vi "UI_page13.vi"(10 "传递队列输入":refnum<queue>, 11 "notifier":refnum<notifier>) -> ()   [LabVIEW 2012]
uses:
  <vilib>/Utility/miscctls.llb/LVDateTimeRec.ctl
  <vilib>/GPower/VIRegister/Library/Convert/ToBool.vi
  <vilib>/GPower/VIRegister/Library/Convert/ToU32.vi
  <vilib>/GPower/VIRegister/Library/Convert/ToU8.vi
  <vilib>/GPower/VIRegister/Library/SubVIs/FindRegisterData.vi
  <vilib>/GPower/VIRegister/Library/SubVIs/ReadSub.vi
  <vilib>/GPower/VIRegister/Library/SubVIs/WriteSub.vi
  <vilib>/GPower/Error/Library/FilterCodes.vi
  <vilib>/GPower/Error/Library/Filter/FilterMulti.vi
  <vilib>/GPower/VIRegister/Library/QManager/GetRegisterData.vi
  <vilib>/GPower/Error/Library/SetError.vi
  <vilib>/GPower/Error/Library/SplitAppended.vi
  <vilib>/GPower/VIRegister/Library/QManager/QManagerAction.vi
  <vilib>/GPower/Error/Library/ErrorType.vi
  <vilib>/GPower/Error/Library/SubVIs/ExplanationToError.vi
  <vilib>/GPower/VIRegister/Library/QManager/GetQName.vi
  <vilib>/GPower/VIRegister/Library/QManager/StartQManager.vi
  <vilib>/Utility/error.llb/Trim Whitespace.vi
  <vilib>/dlg_ctls.llb/Space Constant.vi
  <vilib>/Utility/error.llb/Error Code Database.vi
  <vilib>/GPower/Error/Library/SubVIs/SetStatus.vi
  <vilib>/GPower/Error/Library/AppendErrors.vi
  <vilib>/GPower/Error/Library/Append/AppendSingle.vi
  <vilib>/GPower/VIRegister/VIRegister.lvlib
  <vilib>/measure/NI_MABase.lvlib
panel:
  out "试验已用时":timestamp=timestamp(-28800 s since 1904-01-01) format="%<%H:%M:%S>T"
  in  "测试时间设定":timestamp=timestamp(-28800 s since 1904-01-01) format="%<%H:%M:%S>T"
  in  "停止测量":bool
  in  "开始测量":bool
  out "温度":string
  out "脉冲计数":string
  out "主份G3陀螺脉冲计数":dbl(graph)
  out "主份A3加速度计脉冲计数":dbl(graph)
  out "主份G2陀螺脉冲数":dbl(graph)
  out "主份A2加速度计脉冲计数":dbl(graph)
  out "主份G1陀螺脉冲数":dbl(graph)
  out "主份A1加速度计脉冲计数":dbl(graph)
  out "正确帧计数":u16
  out "错误帧计数":u32
  in  "加计大小量程":enum32{"小量程", "大量程"}(radio)=enum."大量程"
  in  "穿插错误":bool
  in  "少数据字":bool
  in  "少验和":bool
  in  "少帧头":bool
  in  "验和错":bool
  in  "帧头错":bool
  in  "无数据":bool
  in  "地检按钮":bool
  in  "加表频率":dbl=1.0 min=0.1 max=10.0 step=0.1
  in  "加表幅值":dbl=1.0
  in  "陀螺频率":dbl=1.0 min=0.1 max=10.0 step=0.1
  in  "陀螺幅值":dbl=1.0
  # "备  份"
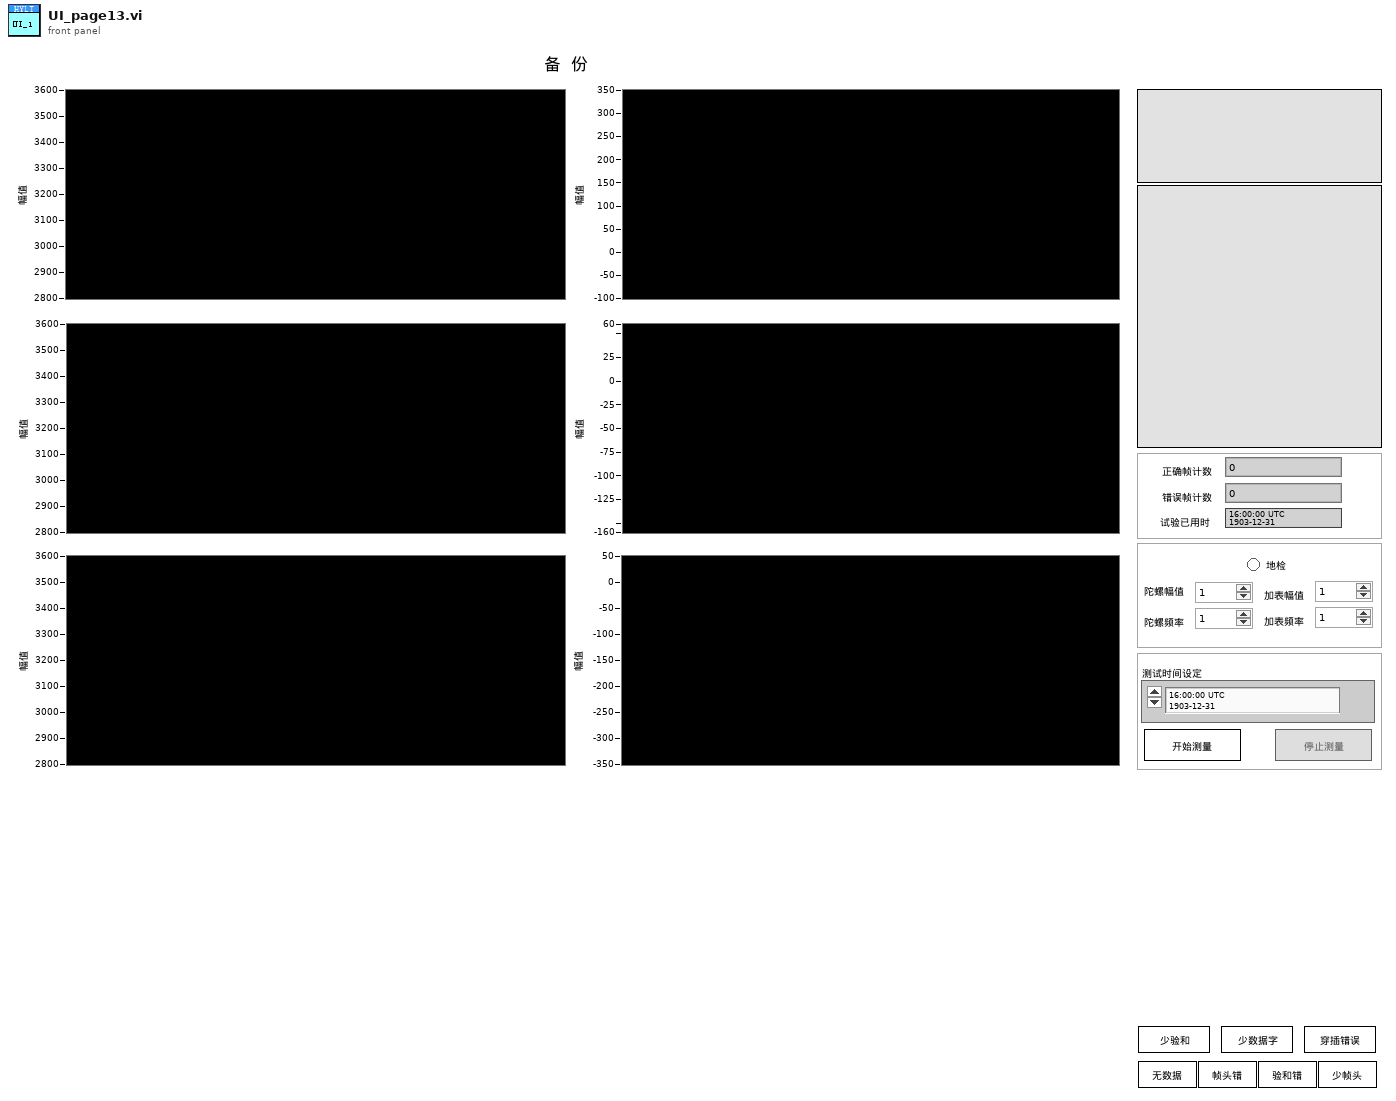
[diagram p1: front panel]
types:
  T1 = typedef "LVDateTimeRec.ctl" = cluster{"fractional second":dbl, "second":i32, "minute":i32, "hour":i32, "day of month":i32, "month":i32, "year":i32, "day of week":i32, "day of year":i32, "DST":i32}
  T2 = enum8{"Enabled", "Disabled", "Disabled and Grayed Out"}
  T3 = enum32{"invalid app kind", "Development System", "Run Time System", "Student Edition", "Embedded LabVIEW", "Evaluation", "Custom"}
  T4 = enum32{"Invalid", "Standard", "Closed", "Hidden", "Minimized", "Maximized"}
  T5 = cluster{"Core":cluster{"Current VI Reference":refnum<vi>, "Close Panel on Exit?":bool}, "传递队列输入":refnum<queue>, "信息帧":cluster{" 数据帧名称":string, " 数据":string, "备用操作符":bool, "起始地址":i32, "读写标志":i32, "长度":i32}, "主份控制指令":u16, "备份控制指令":u16, "notifier ":refnum<notifier>, "秒计数":i64, "起始时间":i64, "定时控制":bool}
  T6 = cluster{" 数据帧名称":string, " 数据":string, "备用操作符":bool, "起始地址":i32, "读写标志":i32, "长度":i32}
  T7 = cluster{"Current VI Reference":refnum<vi>, "Close Panel on Exit?":bool}
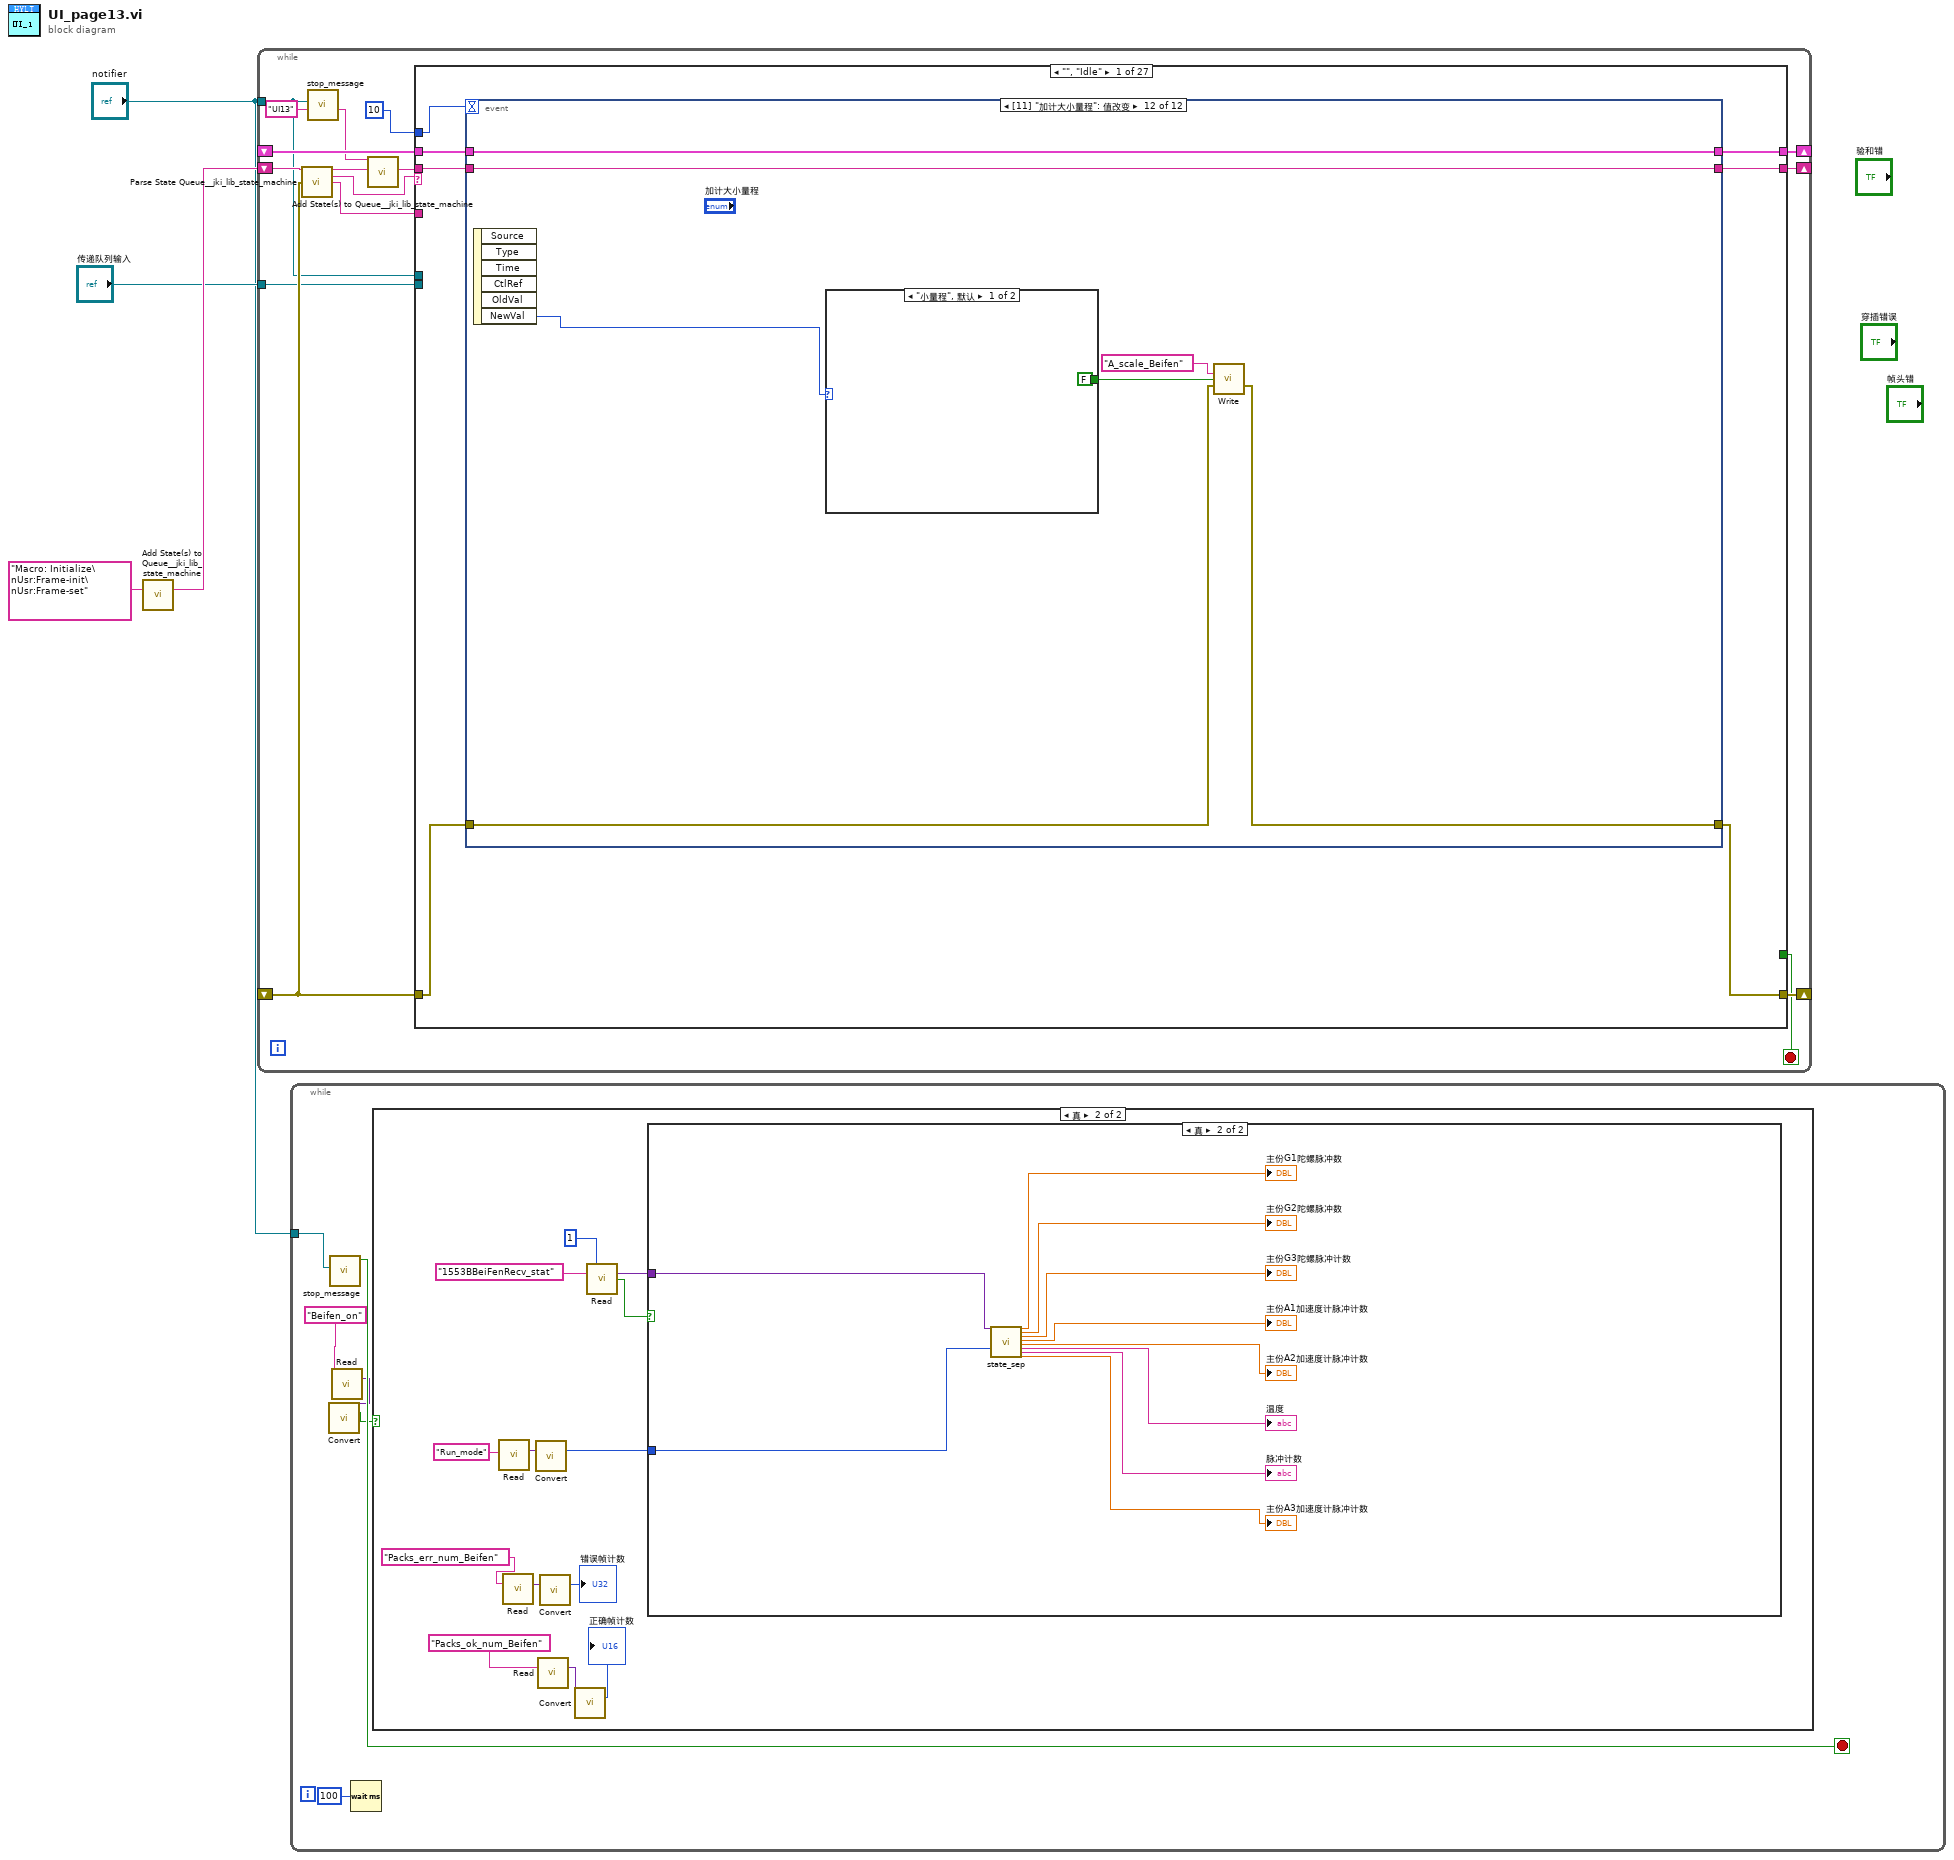
[diagram p0: block diagram]
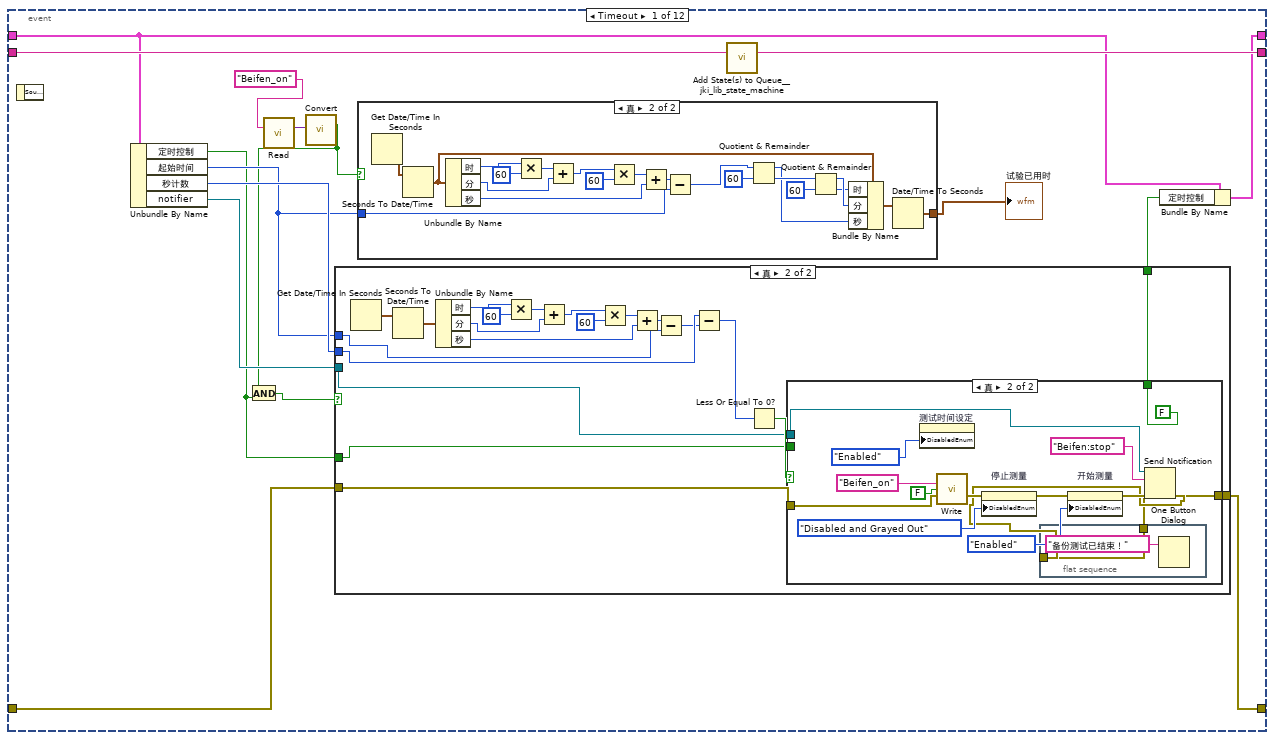
[diagram p4: hidden frame]
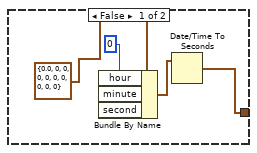
[diagram p5: hidden frame]
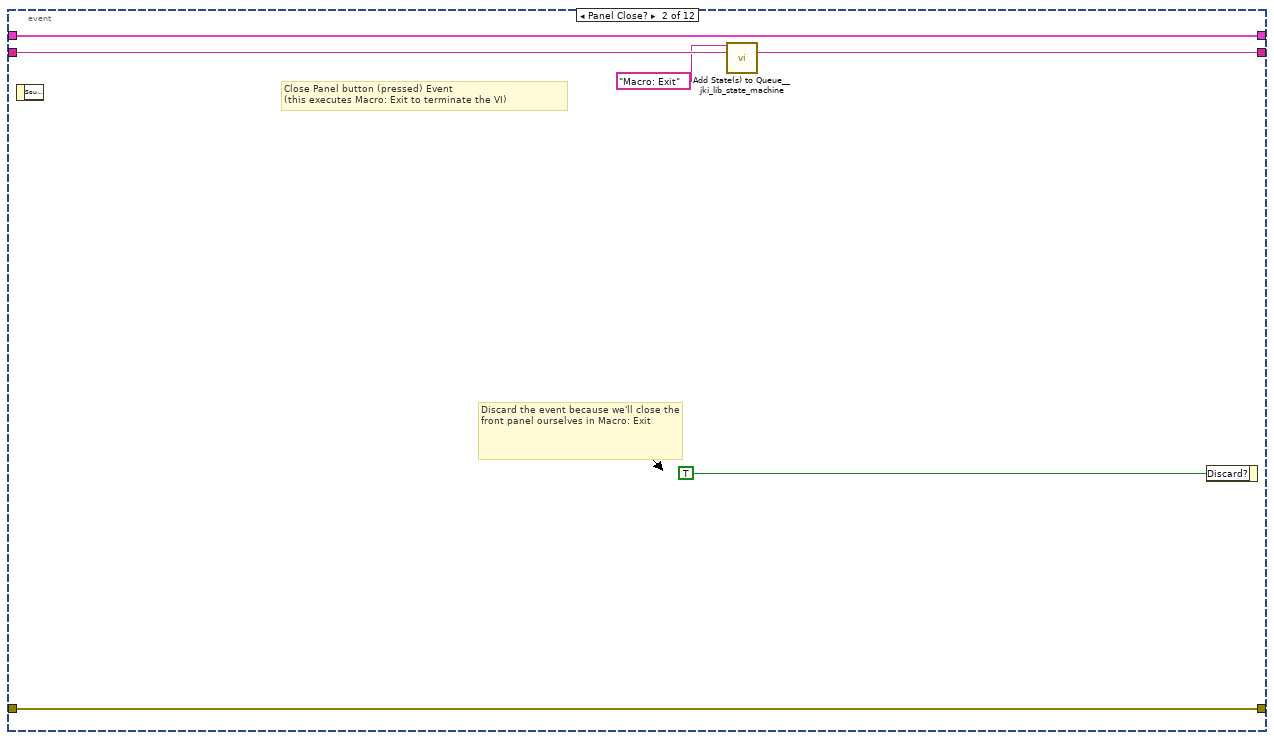
[diagram p8: hidden frame]
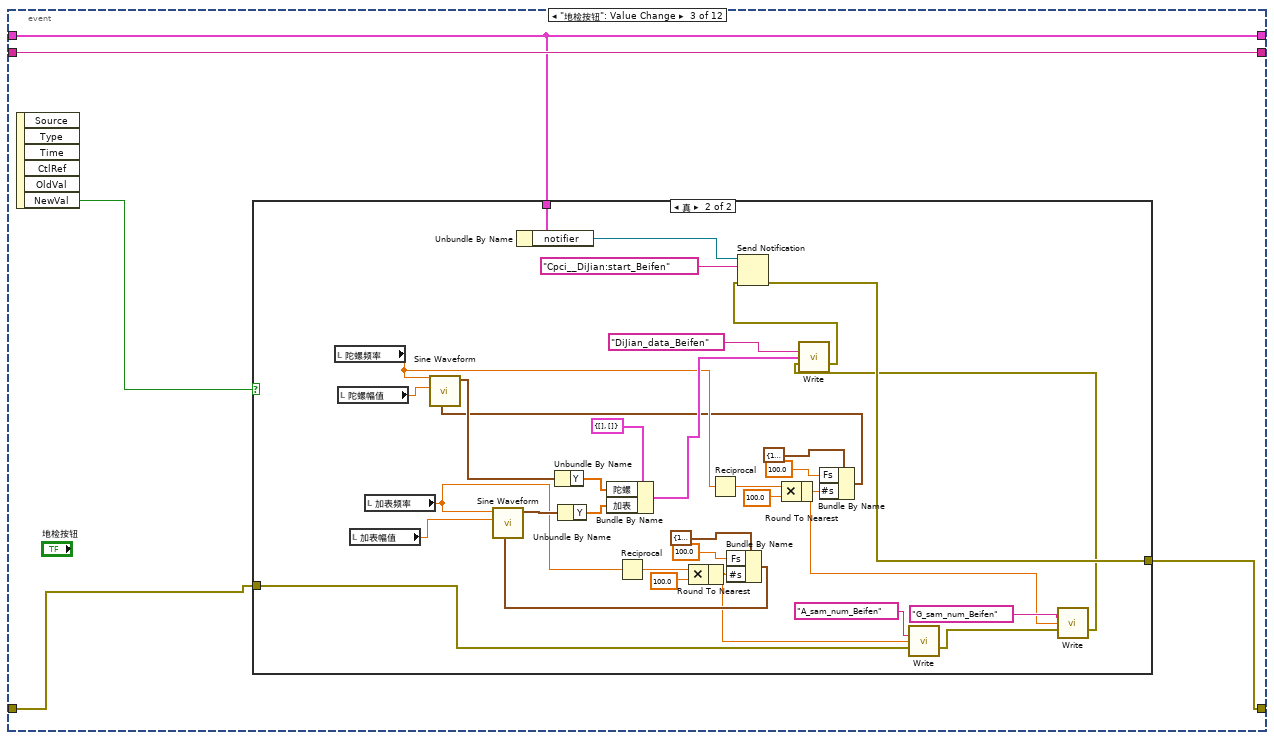
[diagram p9: hidden frame]
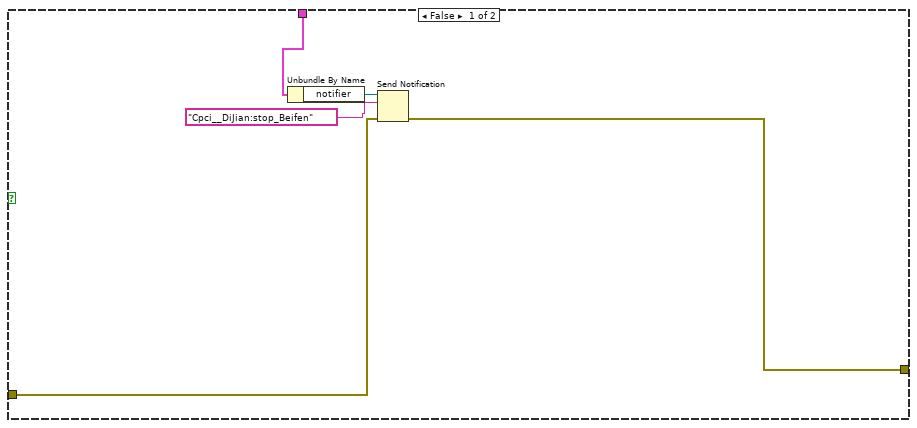
[diagram p10: hidden frame]
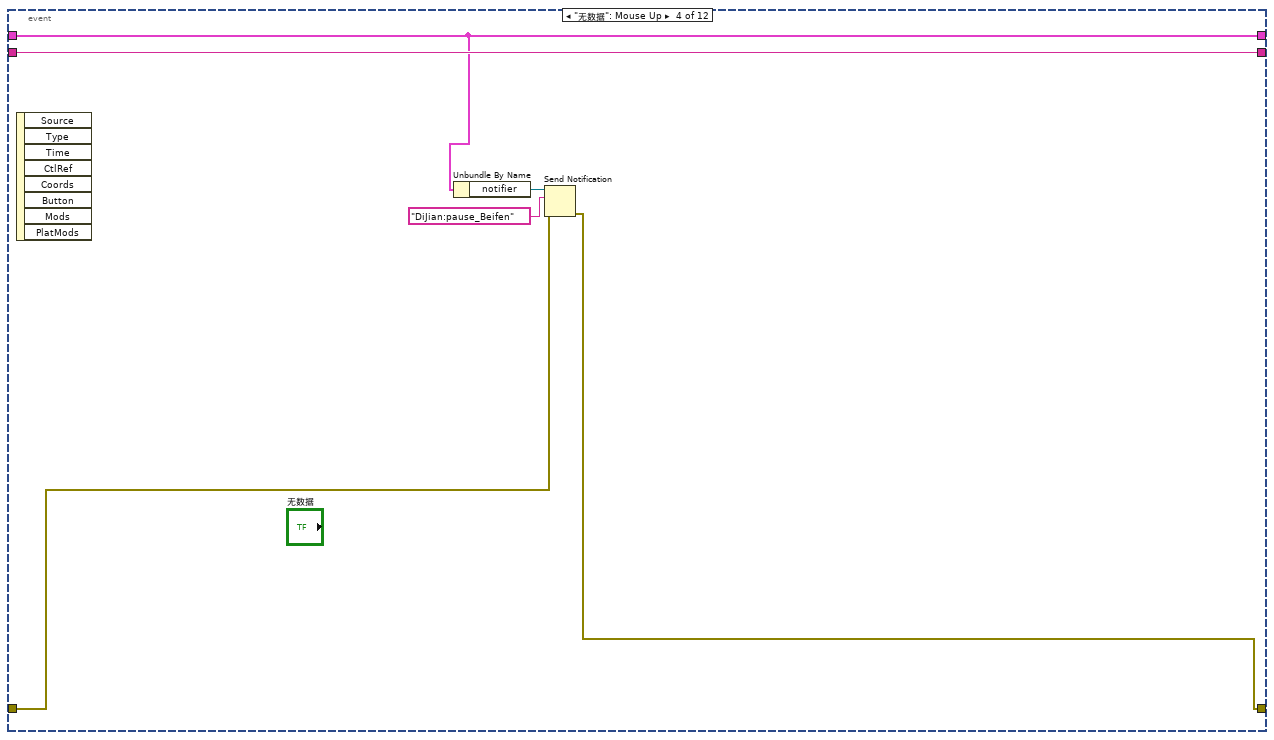
[diagram p11: hidden frame]
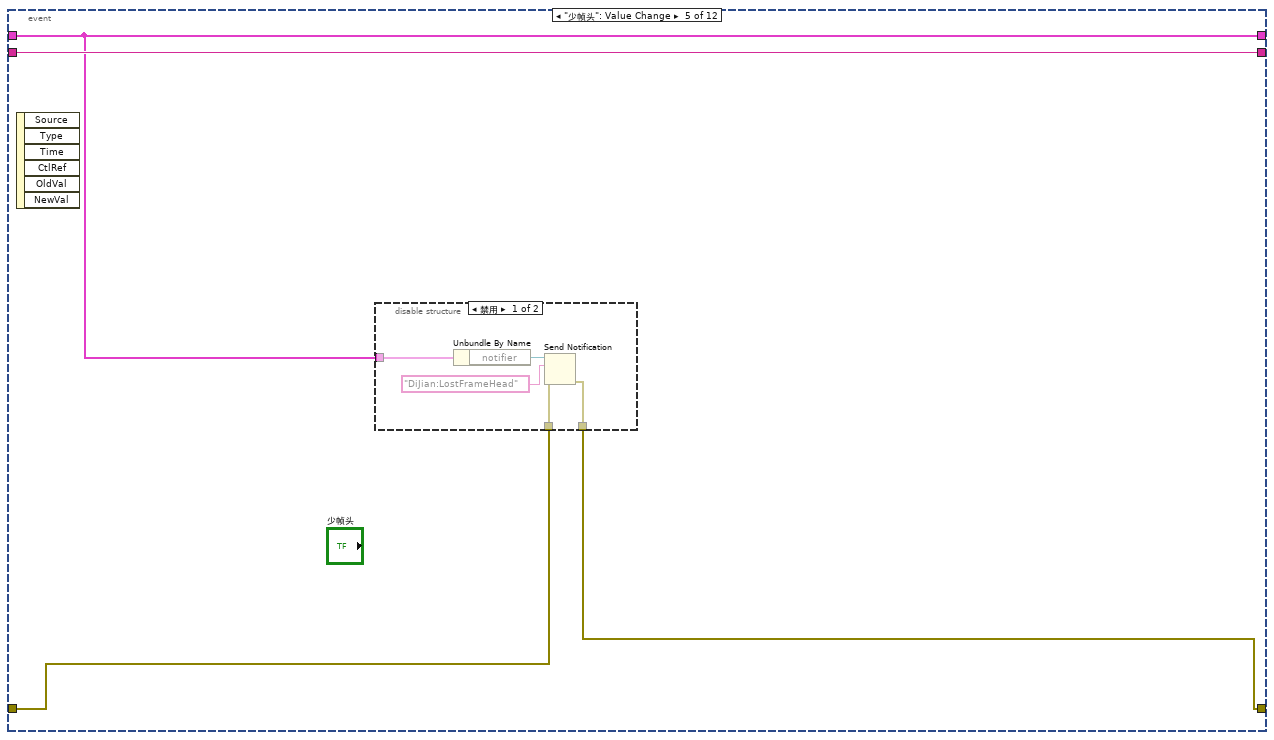
[diagram p12: hidden frame]
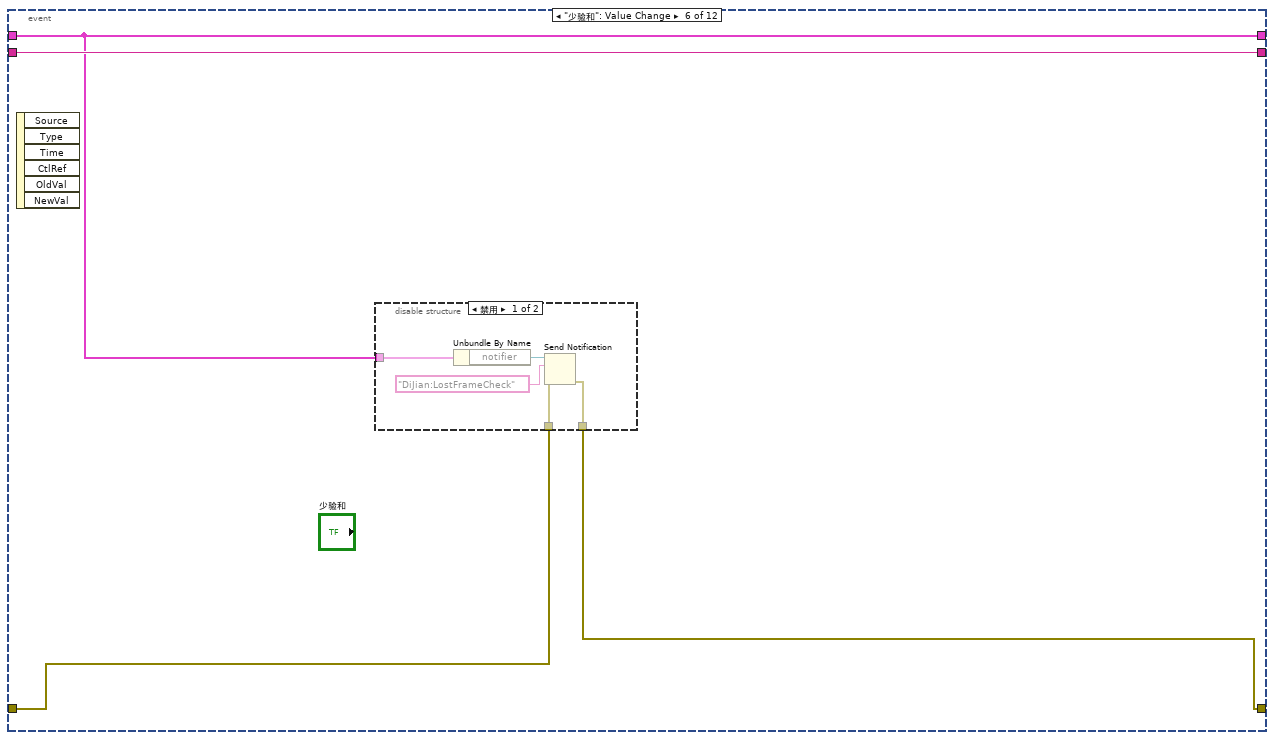
[diagram p14: hidden frame]
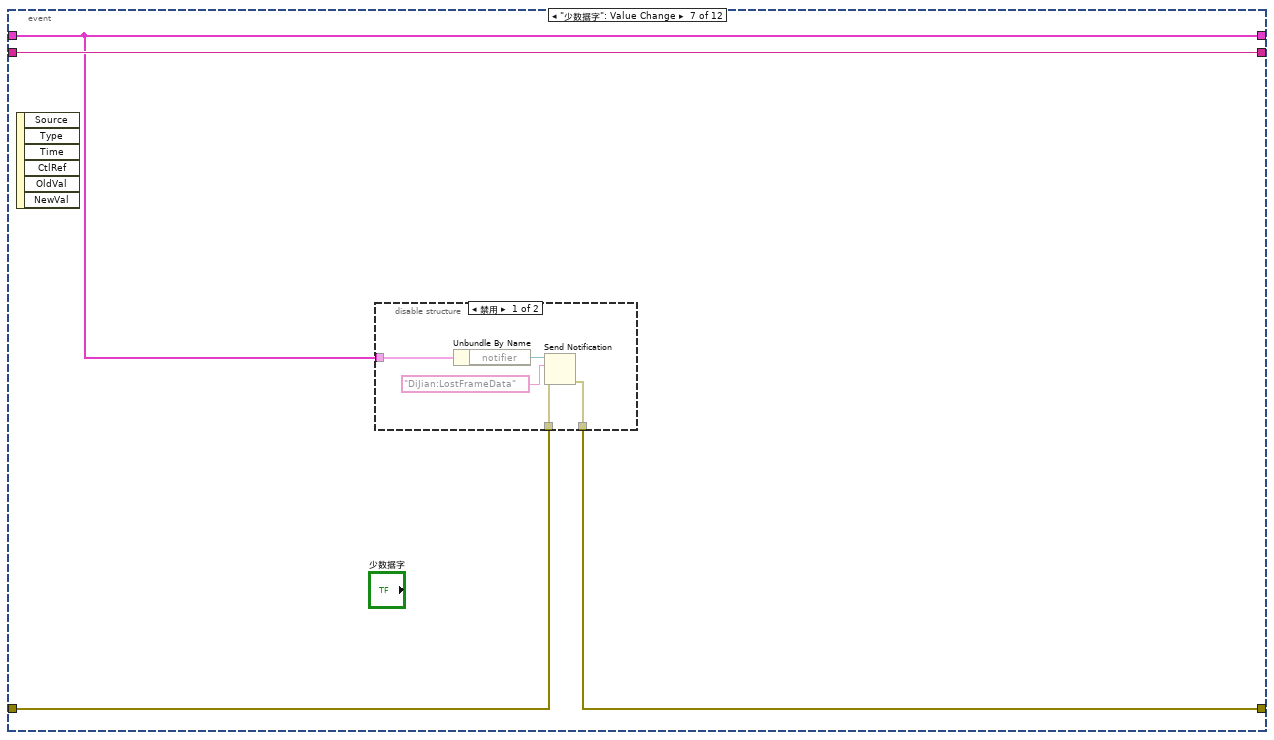
[diagram p16: hidden frame]
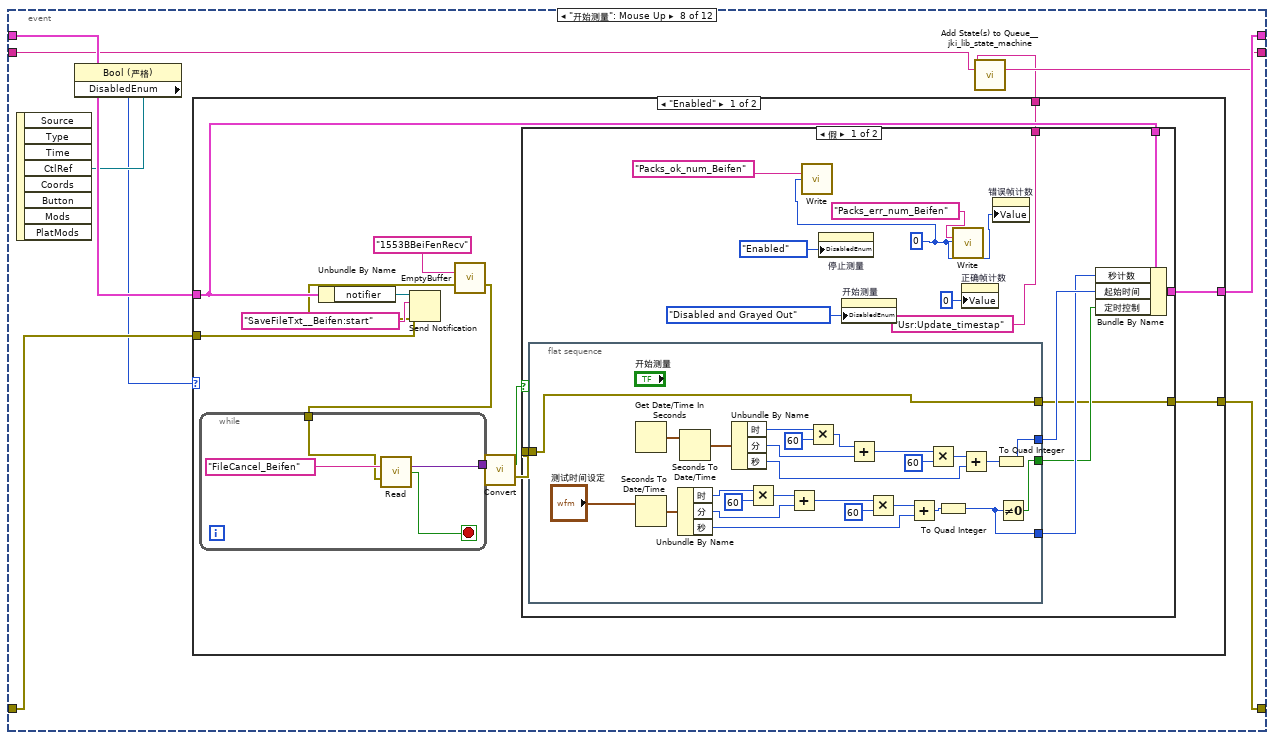
[diagram p18: hidden frame]
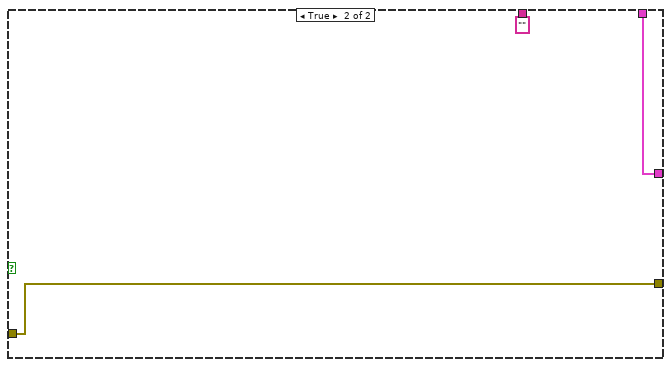
[diagram p19: hidden frame]
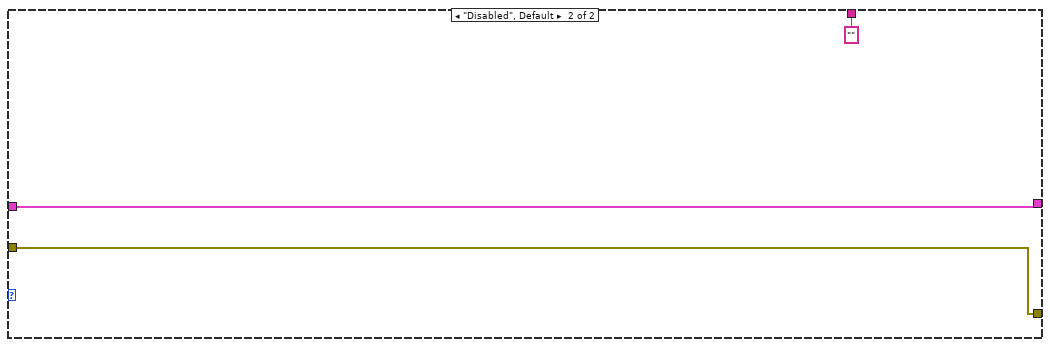
[diagram p20: hidden frame]
diagram:
  n1 = call <vilib>:"Add State(s) to Queue__jki_lib_state_machine.vi"("State(s) in (\"\")"="Macro: Initialize\nUsr:Frame-init\nUsr:Frame-set") -> ("States Out"=w4:string)  [unwired: 14 in]
  n2 = while "JKI - String-Based Queued State Machine (Basic) v1.0" {
    shift-right: [w14] -> _
    shift-left: _ -> [w13]
    shift-right: [w17] -> _
    shift-left: _ -> [w11]
    shift-right: [w16] -> _
    shift-left: w4 -> [w18]
    tunnel: "notifier" -> [w6]
    tunnel: "传递队列输入" -> [w7]
    stop <- w15 stop-if-true
    n3 = call <vilib>:"Parse State Queue__jki_lib_state_machine.vi"("State Queue"=w18, "Error In (no error)"=w11) -> ("Remaining States"=w10:string, "Current State"=w20:string, "Arguments"=w19:string)  [unwired: 11 in]
    n4 = call "stop_message.vi"("识别符"="UI13", "notifier"=w6) -> ("通知"=w9:string)  [unwired: 8 in, 1 out]
    n5 = call <vilib>:"Add State(s) to Queue__jki_lib_state_machine.vi"("State(s) in Front (\"\")"=w9, "State(s) in (\"\")"=w10) -> ("States Out"=w8:string)  [unwired: 13 in]
    n6 = case shown="\"\", \"Idle\"" w20 {
      selector: w20 -> [_ _ w353 _ _ _ _ _ _ _ _ _ _ _ _ _ _ _ _ _ _ _ _ _ _ _ _]
      tunnel: w8 -> [w21 w352 w357 w375 w381 w386 w390 w406 w412 w416 w425 w431 w441 w473 w478 w488 w492 w499 w519 w539 w558 w584 w600 w605 w610 w622 w640]
      tunnel: w19 -> [_ _ _ _ _ _ _ _ _ _ _ w426 w436 _ _ _ _ w493 w513 w533 _ _ _ _ _ _ _]
      tunnel: w13 -> [w26 w349 w355 w366 w378 w384 w387 _ w407 w413 w423 w429 w437 w470 w475 w485 w489 w497 w517 w537 w556 w582 w597 w602 w607 w618 w627]
      tunnel: [w25 w350 w359 w372 errorcluster {"status"=FALSE, "code"=0, "source"=""} ("error out") w383 w388 w403 w408 w414 w422 w427 w438 w471 w476 w486 w490 w495 w515 w535 w554 w580 w598 w603 w608 w620 w625] -> w17
      tunnel: w11 -> [w24 w350 w358 w372 w377 w383 w388 w403 w409 w414 w422 w428 w439 w471 w476 w486 w490 w496 w516 w536 w555 w581 w598 w603 w608 w620 w625]
      tunnel: [w27 w351 w356 w374 w380 w385 w389 w405 w411 w415 w424 w430 w440 w472 w477 w487 w491 w498 w518 w538 w557 w583 w599 w604 w609 w621 w639] -> w16
      tunnel: [_ _ _ _ _ TRUE _ _ _ _ _ _ _ _ _ _ _ _ _ _ _ _ _ _ _ _ _] -> w15
      tunnel: [w23 w349 w355 w373 w378 w384 w387 w404 w407 w413 w423 w429 w437 w470 w475 w485 w489 w494 w514 w534 w553 w579 w597 w602 w606 w618 w626] -> w14
      tunnel: 10 ("Timeout") -> [w22 _ _ _ _ _ _ _ _ _ _ _ _ _ _ _ _ _ _ _ _ _ _ _ _ _ _]
      tunnel: w7 -> [_ _ _ _ _ _ _ w400 _ _ _ _ _ _ _ _ _ _ _ _ _ _ _ _ _ _ _]
      tunnel: w6 -> [_ _ _ _ _ _ _ w396 _ _ _ _ _ _ _ _ _ _ _ _ _ _ _ _ _ _ _]
      frame "", "Idle" {
        n7 = event shown="[11] \"加计大小量程\": 值改变" {
          selector: _ -> [_ _ _ _ _ _ _ _ _ _ _ _]
          dyn-events: _ -> [_ _ _ _ _ _ _ _ _ _ _ _]
          timeout: w22 -> [_ _ _ _ _ _ _ _ _ _ _ _]
          tunnel: w21 -> [w43 w115 w120 w166 w170 w179 w188 w196 w272 w307 w338 w340]
          tunnel: [w42 w114 w120 w166 w170 w179 w188 w195 w272 w307 w338 w340] -> w27
          tunnel: w26 -> [w37 w112 w119 w165 w169 w178 w187 w201 w269 w294 w339 w341]
          tunnel: [w38 w113 w117 w163 w167 w176 w185 w199 w270 w306 w335 w342] -> w25
          tunnel: w24 -> [w39 w113 w118 w164 w168 w177 w186 w202 w271 w306 w334 w343]
          tunnel: [w36 w112 w119 w165 w169 w178 w187 w200 w268 w293 w339 w341] -> w23
          event Timeout {
            n8 = event-data() -> ()  [unwired: 1 in, 1 out]
            n9 = Unbundle By Name(w37) -> ("定时控制"=w28:bool, "起始时间"=w34:i64, "秒计数"=w41:i64, "notifier"=w40:refnum<notifier>)
            n10 = call <vilib>:"Read.vi"("Register name"="Beifen_on") -> ("Register value"=w31:variant)  [unwired: 11 in, 3 out]
            n11 = call-poly <vilib>:"Convert.vi"("Register value in"=w31) -> ("Register value out"=w30:bool)  [unwired: 13 in, 1 out]
            n12 = And(x=w30, y=w28) -> (x .and. y?=w29:bool)
            n13 = case shown="真" w29 {
              tunnel: w34 -> [_ w82]
              tunnel: w41 -> [_ w81]
              tunnel: w40 -> [_ w75]
              tunnel: w39 -> [w70 w74]
              tunnel: [w70 w73] -> w38
              tunnel: [w69 w72] -> w35
              tunnel: w28 -> [w69 w71]
              frame False {
              }
              frame True {
                n14 = Get Date/Time In Seconds() -> (seconds since 1Jan1904=w78:timestamp)
                n15 = Seconds To Date/Time(time stamp (now)=w78) -> (date time rec=w79:T1)  [unwired: 1 in]
                n16 = Unbundle By Name(w79) -> ("时"=w84:i32, "分"=w87:i32, "秒"=w91:i32)
                n17 = Multiply(x=w84, y=60) -> (x*y=w86:i32)
                n18 = Add(x=w86, y=w87) -> (x+y=w88:i32)
                n19 = Multiply(x=w88, y=60) -> (x*y=w90:i32)
                n20 = Add(x=w90, y=w91) -> (x+y=w83:i32)
                n21 = Subtract(x=w83, y=w82) -> (x-y=w80:i64)
                n22 = Subtract(x=w81, y=w80) -> (x-y=w77:i64)
                n23 = Less Or Equal To 0?(x=w77) -> (x <= 0?=w76:bool)
                n24 = case shown="真" w76 {
                  tunnel: w75 -> [_ w99]
                  tunnel: w74 -> [w93 w98]
                  tunnel: [w93 w94] -> w73
                  tunnel: [w92 FALSE] -> w72
                  tunnel: w71 -> [w92 _]
                  frame False {
                  }
                  frame True {
                    n25 = property on="测试时间设定" class="AbsTime (严格)"("DisabledEnum"=T2."Enabled" ("禁用")) -> ()  [unwired: 2 in, 2 out]
                    n26 = call <vilib>:"Write.vi"("Register name"="Beifen_on", "Register value"=FALSE ("停止测量"), "Error in"=w98) -> ("Error out"=w101:errorcluster)  [unwired: 10 in, 2 out]
                    n27 = property on="停止测量" class="Bool (严格)"(error in=w101, "DisabledEnum"=T2."Disabled and Grayed Out" ("禁用")) -> (error out=w102:errorcluster)  [unwired: 1 in, 1 out]
                    n28 = flat-sequence {
                      tunnel: w95 -> [w108]
                      tunnel: [w108] -> w94
                      frame #0 {
                        n29 = One Button Dialog(message="备份测试已结束！" ("消息")) -> ()  [unwired: 1 in, 1 out]
                      }
                    }
                    n30 = property on="开始测量" class="Bool (严格)"(error in=w102, "DisabledEnum"=T2."Enabled" ("禁用")) -> (error out=w100:errorcluster)  [unwired: 1 in, 1 out]
                    n31 = Send Notification(notification="Beifen:stop" ("通知"), notifier=w99, error in (no error)=w100) -> (error out=w95:errorcluster)  [unwired: 1 out]
                  }
                }
              }
            }
            n32 = case shown="真" w30 {
              tunnel: w34 -> [_ w58]
              tunnel: [w44 w50] -> w33
              frame False {
                w46 = 0 ("时")
                n33 = Bundle By Name(cluster=T1 {"fractional second"=0.0, "second"=0, "minute"=0, "hour"=0, "day of month"=0, "month"=0, "year"=0, "day of week"=0, "day of year"=0, "DST"=0} ("日期时间记录 2"), "hour"=w46, "minute"=w46, "second"=w46) -> (w47:T1)
                n34 = Date/Time To Seconds(2:w47) -> (0:w44:timestamp)  [unwired: 1 in]
              }
              frame True {
                n35 = Get Date/Time In Seconds() -> (seconds since 1Jan1904=w68:timestamp)
                n36 = Seconds To Date/Time(time stamp (now)=w68) -> (date time rec=w51:T1)  [unwired: 1 in]
                n37 = Unbundle By Name(w51) -> ("时"=w66:i32, "分"=w63:i32, "秒"=w59:i32)
                n38 = Multiply(x=w66, y=60) -> (x*y=w64:i32)
                n39 = Add(x=w64, y=w63) -> (x+y=w62:i32)
                n40 = Multiply(x=w62, y=60) -> (x*y=w60:i32)
                n41 = Add(x=w60, y=w59) -> (x+y=w67:i32)
                n42 = Subtract(x=w67, y=w58) -> (x-y=w48:i64)
                n43 = Quotient & Remainder(x=w48, y=60) -> (x-y*floor(x/y)=w49:i64, floor(x/y)=w53:i64)
                n44 = Quotient & Remainder(x=w53, y=60) -> (x-y*floor(x/y)=w56:i64, floor(x/y)=w55:i64)
                n45 = Bundle By Name(cluster=w51, "时"=w55, "分"=w56, "秒"=w49) -> (w57:T1)
                n46 = Date/Time To Seconds(2:w57) -> (0:w50:timestamp)  [unwired: 1 in]
              }
            }
            "试验已用时" <- w33
            n47 = call <vilib>:"Add State(s) to Queue__jki_lib_state_machine.vi"("State(s) in (\"\")"=w43) -> ("States Out"=w42:string)  [unwired: 14 in]
            n48 = Bundle By Name(cluster=w37, "定时控制"=w35) -> (w36:T5)
          }
          event Panel Close? {
            # "Discard the event because we'll close the front panel ourselves in Macro: Exit"
            # "Close Panel button (pressed) Event\n(this executes Macro: Exit to terminate the VI)"
            n49 = event-data() -> ()  [unwired: 1 in, 1 out]
            n50 = call <vilib>:"Add State(s) to Queue__jki_lib_state_machine.vi"("State(s) in Front (\"\")"="Macro: Exit", "State(s) in (\"\")"=w115) -> ("States Out"=w114:string)  [unwired: 13 in]
            n51 = event-data("Discard?"=TRUE) -> ()  [unwired: 1 in, 1 out]
          }
          event "地检按钮": Value Change {
            n52 = event-data() -> ("NewVal"=w116:bool)  [unwired: 1 in, 5 out]
            n53 = case shown="真" w116 {
              tunnel: [w121 w147] -> w117
              tunnel: w119 -> [w123 w157]
              tunnel: w118 -> [w122 w127]
              frame False {
                n54 = Unbundle By Name(w123) -> ("notifier"=w124:refnum<notifier>)
                n55 = Send Notification(notification="Cpci__DiJian:stop_Beifen" ("通知"), notifier=w124, error in (no error)=w122) -> (error out=w121:errorcluster)  [unwired: 1 out]
              }
              frame True {
                n56 = local read "陀螺频率"() -> (w136:dbl)
                n57 = local read "陀螺幅值"() -> (w149:dbl)
                n58 = local read "加表幅值"() -> (w150:dbl)
                n59 = local read "加表频率"() -> (w142:dbl)
                n60 = Unbundle By Name(w157) -> ("notifier"=w158:refnum<notifier>)
                n61 = Reciprocal(x=w142) -> (1/x=w146:dbl)
                n62 = Multiply(x=w146, y=100.0) -> (x*y=w133:dbl)
                n63 = Round To Nearest(number=w133) -> (nearest integer value=w128:dbl)
                n64 = Reciprocal(x=w136) -> (1/x=w140:dbl)
                n65 = Bundle By Name(cluster=cluster{"Fs":dbl, "#s":dbl} {"Fs"=1000.0, "#s"=1000.0} ("sampling info"), "Fs"=100.0, "#s"=w128) -> (w141:cluster{"Fs":dbl, "#s":dbl})
                n66 = call <vilib>:"Sine Waveform.vi"("sampling info"=w141, "amplitude"=w150, "frequency"=w142) -> ("signal out"=w154:waveform(dbl))  [unwired: 7 in, 1 out]
                n67 = Unbundle By Name(w154) -> ("Y"=w152:dbl[])
                n68 = Multiply(x=w140, y=100.0) -> (x*y=w131:dbl)
                n69 = Round To Nearest(number=w131) -> (nearest integer value=w129:dbl)
                n70 = Bundle By Name(cluster=cluster{"Fs":dbl, "#s":dbl} {"Fs"=1000.0, "#s"=1000.0} ("sampling info"), "Fs"=100.0, "#s"=w129) -> (w135:cluster{"Fs":dbl, "#s":dbl})
                n71 = call <vilib>:"Sine Waveform.vi"("sampling info"=w135, "amplitude"=w149, "frequency"=w136) -> ("signal out"=w155:waveform(dbl))  [unwired: 7 in, 1 out]
                n72 = Unbundle By Name(w155) -> ("Y"=w151:dbl[])
                n73 = Bundle By Name(cluster=cluster{"陀螺":dbl[], "加表":dbl[]} {"陀螺"=[], "加表"=[]} ("输入簇"), "陀螺"=w151, "加表"=w152) -> (w156:cluster{"陀螺":dbl[], "加表":dbl[]})
                n74 = call <vilib>:"Write.vi"("Register name"="A_sam_num_Beifen", "Register value"=w128, "Error in"=w127) -> ("Error out"=w130:errorcluster)  [unwired: 10 in, 2 out]
                n75 = call <vilib>:"Write.vi"("Register name"="G_sam_num_Beifen", "Register value"=w129, "Error in"=w130) -> ("Error out"=w126:errorcluster)  [unwired: 10 in, 2 out]
                n76 = call <vilib>:"Write.vi"("Register name"="DiJian_data_Beifen", "Register value"=w156, "Error in"=w126) -> ("Error out"=w148:errorcluster)  [unwired: 10 in, 2 out]
                n77 = Send Notification(notification="Cpci__DiJian:start_Beifen" ("通知"), notifier=w158, error in (no error)=w148) -> (error out=w147:errorcluster)  [unwired: 1 out]
              }
            }
          }
          event "无数据": Mouse Up {
            n78 = event-data() -> ()  [unwired: 1 in, 8 out]
            n79 = Unbundle By Name(w165) -> ("notifier"=w161:refnum<notifier>)
            n80 = Send Notification(notification="DiJian:pause_Beifen" ("通知"), notifier=w161, error in (no error)=w164) -> (error out=w163:errorcluster)  [unwired: 1 out]
          }
          event "少帧头": Value Change {
            n81 = event-data() -> ()  [unwired: 1 in, 6 out]
            n82 = disable-structure shown="禁用" {
              disable-tunnel: w169 -> [w175 _]
              disable-tunnel: w168 -> [w174 _]
              disable-tunnel: [w173 _] -> w167
              frame Disabled {
                n83 = Unbundle By Name(w175) -> ("notifier"=w171:refnum<notifier>)
                n84 = Send Notification(notification="DiJian:LostFrameHead" ("通知"), notifier=w171, error in (no error)=w174) -> (error out=w173:errorcluster)  [unwired: 1 out]
              }
              frame Enabled {
              }
            }
          }
          event "少验和": Value Change {
            n85 = event-data() -> ()  [unwired: 1 in, 6 out]
            n86 = disable-structure shown="禁用" {
              disable-tunnel: w178 -> [w184 _]
              disable-tunnel: w177 -> [w183 _]
              disable-tunnel: [w182 _] -> w176
              frame Disabled {
                n87 = Unbundle By Name(w184) -> ("notifier"=w180:refnum<notifier>)
                n88 = Send Notification(notification="DiJian:LostFrameCheck" ("通知"), notifier=w180, error in (no error)=w183) -> (error out=w182:errorcluster)  [unwired: 1 out]
              }
              frame Enabled {
              }
            }
          }
          event "少数据字": Value Change {
            n89 = event-data() -> ()  [unwired: 1 in, 6 out]
            n90 = disable-structure shown="禁用" {
              disable-tunnel: w187 -> [w193 _]
              disable-tunnel: w186 -> [w192 _]
              disable-tunnel: [w191 _] -> w185
              frame Disabled {
                n91 = Unbundle By Name(w193) -> ("notifier"=w189:refnum<notifier>)
                n92 = Send Notification(notification="DiJian:LostFrameData" ("通知"), notifier=w189, error in (no error)=w192) -> (error out=w191:errorcluster)  [unwired: 1 out]
              }
              frame Enabled {
              }
            }
          }
          event "开始测量": Mouse Up {
            n93 = event-data() -> ("CtlRef"=w198:refnum<vi>)  [unwired: 1 in, 7 out]
            n94 = property class="Bool (严格)"(reference=w198) -> ("DisabledEnum"=w197:T2)  [unwired: 1 in, 2 out]
            n95 = case shown="\"Enabled\"" w197 {
              tunnel: w202 -> [w213 w264]
              tunnel: w201 -> [w212 w265]
              tunnel: [w211 w265] -> w200
              tunnel: [w210 w264] -> w199
              tunnel: [w203 "" ("State(s) in Front (\"\")")] -> w194
              frame "Enabled" {
                n96 = Unbundle By Name(w212) -> ("notifier"=w214:refnum<notifier>)
                n97 = Send Notification(notification="SaveFileTxt__Beifen:start" ("通知"), notifier=w214, error in (no error)=w213) -> (error out=w206:errorcluster)  [unwired: 1 out]
                n98 = call <vilib>:"EmptyBuffer.vi"("Register name"="1553BBeiFenRecv", "Error in"=w206) -> ("Error out"=w205:errorcluster)  [unwired: 11 in, 2 out]
                n99 = while {
                  tunnel: w205 -> [w261]
                  tunnel: [w259] -> w209
                  stop <- w260 stop-if-true
                  n100 = call <vilib>:"Read.vi"("Register name"="FileCancel_Beifen", "Error in"=w261) -> ("Register value"=w259:variant, "Register value read?"=w260:bool)  [unwired: 10 in, 2 out]
                }
                n101 = call-poly <vilib>:"Convert.vi"("Register value in"=w209) -> ("Register value out"=w207:bool, "Error out"=w208:errorcluster)  [unwired: 13 in]
                n102 = case shown="假" w207 {
                  tunnel: w212 -> [w227 w257]
                  tunnel: [w224 w257] -> w211
                  tunnel: [w222 w258] -> w210
                  tunnel: w208 -> [w221 w258]
                  tunnel: ["Usr:Update_timestap" ("State(s) in Front (\"\")") "" ("State(s) in Front (\"\")")] -> w203
                  frame False {
                    w218 = u32 0
                    n103 = flat-sequence {
                      tunnel: [w233] -> w226
                      tunnel: [w232] -> w225
                      tunnel: [w231] -> w223
                      tunnel: w221 -> [w230]
                      tunnel: [w230] -> w222
                      frame #0 {
                        n104 = Get Date/Time In Seconds() -> (seconds since 1Jan1904=w245:timestamp)
                        n105 = Seconds To Date/Time(time stamp (now)="测试时间设定") -> (date time rec=w254:T1)  [unwired: 1 in]
                        n106 = Unbundle By Name(w254) -> ("时"=w253:i32, "分"=w250:i32, "秒"=w246:i32)
                        n107 = Seconds To Date/Time(time stamp (now)=w245) -> (date time rec=w236:T1)  [unwired: 1 in]
                        n108 = Unbundle By Name(w236) -> ("时"=w237:i32, "分"=w240:i32, "秒"=w244:i32)
                        n109 = Multiply(x=w253, y=60) -> (x*y=w251:i32)
                        n110 = Add(x=w251, y=w250) -> (x+y=w249:i32)
                        n111 = Multiply(x=w237, y=60) -> (x*y=w239:i32)
                        n112 = Add(x=w239, y=w240) -> (x+y=w241:i32)
                        n113 = Multiply(x=w249, y=60) -> (x*y=w247:i32)
                        n114 = Add(x=w247, y=w246) -> (x+y=w234:i32)
                        n115 = Multiply(x=w241, y=60) -> (x*y=w243:i32)
                        n116 = To Quad Integer(1:w234) -> (0:w232:i64)
                        n117 = Add(x=w243, y=w244) -> (x+y=w235:i32)
                        n118 = To Quad Integer(1:w235) -> (0:w233:i64)
                        n119 = Not Equal To 0?(x=w232) -> (x != 0?=w231:bool)
                      }
                    }
                    n120 = call <vilib>:"Write.vi"("Register name"="Packs_ok_num_Beifen", "Register value"=w218) -> ()  [unwired: 11 in, 3 out]
                    n121 = property on="停止测量" class="Bool (严格)"("DisabledEnum"=T2."Enabled" ("禁用")) -> ()  [unwired: 2 in, 2 out]
                    n122 = property on="开始测量" class="Bool (严格)"("DisabledEnum"=T2."Disabled and Grayed Out" ("禁用")) -> ()  [unwired: 2 in, 2 out]
                    n123 = call <vilib>:"Write.vi"("Register name"="Packs_err_num_Beifen", "Register value"=w218) -> ()  [unwired: 11 in, 3 out]
                    n124 = property on="正确帧计数" class="DigNum (严格)"("Value"=u16 0 ("脉冲  累计")) -> ()  [unwired: 2 in, 2 out]
                    n125 = property on="错误帧计数" class="DigNum (严格)"("Value"=w218) -> ()  [unwired: 2 in, 2 out]
                    n126 = Bundle By Name(cluster=w227, "秒计数"=w225, "起始时间"=w226, "定时控制"=w223) -> (w224:T5)
                  }
                  frame True {
                  }
                }
              }
              frame "Disabled", Default {
              }
            }
            n127 = call <vilib>:"Add State(s) to Queue__jki_lib_state_machine.vi"("State(s) in Front (\"\")"=w194, "State(s) in (\"\")"=w196) -> ("States Out"=w195:string)  [unwired: 13 in]
          }
          event "停止测量": Mouse Up {
            n128 = event-data() -> ("CtlRef"=w267:refnum<vi>)  [unwired: 1 in, 7 out]
            n129 = property class="Bool (严格)"(reference=w267) -> ("DisabledEnum"=w266:T2)  [unwired: 1 in, 2 out]
            n130 = case shown="\"Enabled\"" w266 {
              tunnel: w271 -> [w280 w290]
              tunnel: [w279 w290] -> w270
              tunnel: w269 -> [w277 w289]
              tunnel: [w276 w289] -> w268
              frame "Enabled" {
                n131 = call <vilib>:"Write.vi"("Register name"="Beifen_on", "Register value"=FALSE ("停止测量"), "Error in"=w280) -> ("Error out"=w281:errorcluster)  [unwired: 10 in, 2 out]
                n132 = property on="停止测量" class="Bool (严格)"(error in=w281, "DisabledEnum"=T2."Disabled and Grayed Out" ("禁用")) -> (error out=w282:errorcluster)  [unwired: 1 in, 1 out]
                n133 = property on="开始测量" class="Bool (严格)"(error in=w282, "DisabledEnum"=T2."Enabled" ("禁用")) -> (error out=w274:errorcluster)  [unwired: 1 in, 1 out]
                n134 = Unbundle By Name(w277) -> ("notifier"=w286:refnum<notifier>)
                n135 = property on="测试时间设定" class="AbsTime (严格)"(error in=w274, "DisabledEnum"=T2."Enabled" ("禁用")) -> (error out=w273:errorcluster)  [unwired: 1 in, 1 out]
                n136 = Send Notification(notification="Cpci__Beifen:stop" ("通知"), notifier=w286, error in (no error)=w273) -> (error out=w279:errorcluster)  [unwired: 1 out]
                n137 = Bundle By Name(cluster=w277, "定时控制"=FALSE) -> (w276:T5)
              }
              frame "Disabled", Default {
              }
            }
          }
          event "测试时间设定": Value Change {
            n138 = event-data() -> ("NewVal"=w296:timestamp)  [unwired: 1 in, 5 out]
            n139 = Seconds To Date/Time(time stamp (now)=w296) -> (date time rec=w305:T1)  [unwired: 1 in]
            n140 = Unbundle By Name(w305) -> ("时"=w304:i32, "分"=w301:i32, "秒"=w297:i32)
            n141 = Multiply(x=w304, y=60) -> (x*y=w302:i32)
            n142 = Add(x=w302, y=w301) -> (x+y=w300:i32)
            n143 = Multiply(x=w300, y=60) -> (x*y=w298:i32)
            n144 = Add(x=w298, y=w297) -> (x+y=w292:i32)
            n145 = To Quad Integer(1:w292) -> (0:w295:i64)
            n146 = Not Equal To 0?(x=w292) -> (x != 0?=w291:bool)
            n147 = Bundle By Name(cluster=w294, "秒计数"=w295, "定时控制"=w291) -> (w293:T5)
          }
          event "陀螺幅值", "陀螺频率", "加表幅值", "加表频率": Value Change {
            n148 = event-data() -> ()  [unwired: 1 in, 6 out]
            n149 = Reciprocal(x="陀螺频率") -> (1/x=w320:dbl)
            n150 = Multiply(x=w320, y=100.0) -> (x*y=w310:dbl)
            n151 = Round To Nearest(number=w310) -> (nearest integer value=w308:dbl)
            n152 = Bundle By Name(cluster=cluster{"Fs":dbl, "#s":dbl} {"Fs"=1000.0, "#s"=1000.0} ("sampling info"), "Fs"=100.0, "#s"=w308) -> (w315:cluster{"Fs":dbl, "#s":dbl})
            n153 = call <vilib>:"Sine Waveform.vi"("sampling info"=w315, "amplitude"="陀螺幅值", "frequency"="陀螺频率") -> ("signal out"=w333:waveform(dbl))  [unwired: 7 in, 1 out]
            n154 = Reciprocal(x="加表频率") -> (1/x=w326:dbl)
            n155 = Multiply(x=w326, y=100.0) -> (x*y=w311:dbl)
            n156 = Unbundle By Name(w333) -> ("Y"=w329:dbl[])
            n157 = Round To Nearest(number=w311) -> (nearest integer value=w309:dbl)
            n158 = Bundle By Name(cluster=cluster{"Fs":dbl, "#s":dbl} {"Fs"=1000.0, "#s"=1000.0} ("sampling info"), "Fs"=100.0, "#s"=w309) -> (w321:cluster{"Fs":dbl, "#s":dbl})
            n159 = call <vilib>:"Sine Waveform.vi"("sampling info"=w321, "amplitude"="加表幅值", "frequency"="加表频率") -> ("signal out"=w332:waveform(dbl))  [unwired: 7 in, 1 out]
            n160 = Unbundle By Name(w332) -> ("Y"=w330:dbl[])
            n161 = Bundle By Name(cluster=cluster{"陀螺":dbl[], "加表":dbl[]} {"陀螺"=[], "加表"=[]} ("输入簇"), "陀螺"=w329, "加表"=w330) -> (w336:cluster{"陀螺":dbl[], "加表":dbl[]})
            n162 = call <vilib>:"Write.vi"("Register name"="DiJian_data_Beifen", "Register value"=w336, "Error in"=w334) -> ("Error out"=w335:errorcluster)  [unwired: 10 in, 2 out]
            n163 = call <vilib>:"Write.vi"("Register name"="A_sam_num_Beifen", "Register value"=w309) -> ("Error out"=w312:errorcluster)  [unwired: 11 in, 2 out]
            n164 = call <vilib>:"Write.vi"("Register name"="G_sam_num_Beifen", "Register value"=w308, "Error in"=w312) -> ()  [unwired: 10 in, 3 out]
          }
          event "加计大小量程": Value Change {
            n165 = event-data() -> ("NewVal"=w346:enum32{"小量程", "大量程"})  [unwired: 1 in, 5 out]
            n166 = case shown="\"小量程\", 默认" w346 {
              tunnel: [FALSE TRUE] -> w344
              frame "小量程", Default {
              }
              frame "大量程" {
              }
            }
            n167 = call <vilib>:"Write.vi"("Register name"="A_scale_Beifen", "Register value"=w344, "Error in"=w343) -> ("Error out"=w342:errorcluster)  [unwired: 10 in, 2 out]
          }
        }
      }
      frame "---------- Core ----------" {
        # "Do not put any code in this frame.\n(it is a separator no-op)"
        n168 = call <vilib>:"Add State(s) to Queue__jki_lib_state_machine.vi"("State(s) in (\"\")"=w352) -> ("States Out"=w351:string)  [unwired: 14 in]
      }
      frame Default {
        w362 = 42 items=["No error", "Argument error", "Memory is full", "Out of zone", "End of file", "File already open", "Generic file I/O error", "File not found", "File permission error", "Disk is full", "Duplicate path", "Too many files open", "System feature not enabled", "Resource file not found", "Cannot add resource", "Resource not found", "Image not found", "Image memory error", "Pen does not exist", "Config type invalid", "Config token not found", "Config parse error", "Config memory error", "Bad external code format", "Bad external code offset", "External code not present", "Null window", "Destroy window error", "Null menu", "Print aborted", "Bad print record", "Print driver error", "Windows error during printing", "Memory error during printing", "Print dialog error", "Generic print error", "Invalid device refnum", "Device not found", "Device parameter error", "Device unit error", "Cannot open device", "Device call aborted", "Generic error", "Cancelled by user", "Object ID too low", "Object ID too high", "Object not in heap", "Unknown heap", "Unknown object (invalid DefProc)", "Unknown object (DefProc not in table)", "Message out of range", "Invalid (null) method", "Unknown message", "Manager call not supported", "Bad address", "Network operation in progress", "Network operation timed out", "Connection is busy", "Network attribute not supported", "Network error", "Address in use", "System out of memory", "Connection aborted", "Connection refused", "Not connected", "Already connected", "Connection closed", "Initialization error (interapplication manager)", "Bad occurrence", "Wait on unbound occurrence handler", "Occurrence queue overflow", "Datalog type conflict", "Unused", "Unrecognized type (interapplication manager)", "Memory corrupt", "Failed to make temporary DLL", "Old CIN version", "Drag socket not found", "Failed to load drop-object", "Failed to register OLE object", "Failed to release OLE object", "Format specifier type mismatch", "Unknown format specifier", "Too few format specifiers", "Too many format specifiers", "Scan failed", "Newer CIN version", "Error converting to variant", "Runtime menu error", "Password tampered", "Variant attribute not found", "Incompatible variant data type", "Event data is not available", "Event Store is not present", "Occurrence is not found", "Event Queue is not created", "Event info is not available", "Refnum passed is NULL", "Error retrieving Class GUID", "Error retrieving CoClass GUID", "Error retrieving TypeLib GUID.", "Bad built application magic bytes.", "Specific driver is different from the specific driver associated with the Logical Name.", "There is no session opened to the class driver.", "Max Error", "MAX - Error with config objects", "MAX - Error loading configuration", "MAX - Group not supported"]
        # "Current State"
        # "Do not delete, rename, or modify this frame.\n(this is used to capture unhandled states and typos)"
        # "Handle mistyped state name (developer tool)"
        n169 = Format Into String(format string="Software Exception: Unhandled State \"%s\"." ("message"), error in=w358, w353) -> (resulting string=w361:string, error out=w360:errorcluster)  [unwired: 1 in]
        n170 = call <vilib>:"Error Cluster From Error Code.vi"("show call chain? (False)"=TRUE, "error in (no error)"=w360, "error message (\"\")"=w361, "error code (0)"=w362) -> ("error out"=w359:errorcluster)  [unwired: 5 in]
        n171 = call <vilib>:"Add State(s) to Queue__jki_lib_state_machine.vi"("State(s) in (\"\")"=w357) -> ("States Out"=w356:string)  [unwired: 14 in]
      }
      frame "Initialize Core Data" {
        # "Do not delete, rename, or modify this frame.\n(this is used to determine panel behavior on exit)"
        # "originally closed?"
        # "exe?"
        # "If panel starts closed or is an EXE, then close it when we exit"
        n172 = property class="VI"() -> ("Front Panel.Open"=w371:bool)  [unwired: 2 in, 2 out]
        n173 = property class="App"() -> ("App.Kind"=w370:T3)  [unwired: 2 in, 2 out]
        n174 = control-ref of="Current VI Reference"() -> (w364:refnum<vi>)
        n175 = Not(x=w371) -> (.not. x?=w368:bool)
        n176 = Equal?(x=w370, y=T3."Run Time System" ("Application:Kind")) -> (x = y?=w367:bool)
        n177 = Or(x=w368, y=w367) -> (x .or. y?=w365:bool)
        n178 = Bundle By Name(cluster=w366, "Core.Current VI Reference"=w364, "Core.Close Panel on Exit?"=w365) -> (w373:T5)
        n179 = call <vilib>:"Add State(s) to Queue__jki_lib_state_machine.vi"("State(s) in (\"\")"=w375) -> ("States Out"=w374:string)  [unwired: 14 in]
      }
      frame "Error Handler" {
        # "Unhandled Error -- Display it"
        # "Handle any errors here.\nYou can also output any states to clean-up after errors occur"
        # "Clear error"
        n180 = call <vilib>:"General Error Handler.vi"("error in (no error)"=w377) -> ()  [unwired: 10 in, 5 out]
        n181 = call <vilib>:"Add State(s) to Queue__jki_lib_state_machine.vi"("State(s) in Front (\"\")"="/* Post Error States", "State(s) in (\"\")"=w381) -> ("States Out"=w380:string)  [unwired: 13 in]
      }
      frame "Exit" {
        n182 = call <vilib>:"Add State(s) to Queue__jki_lib_state_machine.vi"("State(s) in (\"\")"=w386) -> ("States Out"=w385:string)  [unwired: 14 in]
      }
      frame "---------- Data ----------" {
        # "Do not put any code in this frame.\n(It is a separator no-op. You can make a copy of this frame to create a new Data frame)"
        n183 = call <vilib>:"Add State(s) to Queue__jki_lib_state_machine.vi"("State(s) in (\"\")"=w390) -> ("States Out"=w389:string)  [unwired: 14 in]
      }
      frame "Data: Initialize" {
        w393 = FALSE  # 定时控制
        w394 = i64 0  # 起始时间
        w395 = i64 0  # 秒计数
        w392 = FALSE
        w398 = u16 0  # 备份控制指令
        w399 = u16 0  # 主份控制指令
        w401 = T6 {" 数据帧名称"="", " 数据"="", "备用操作符"=TRUE, "起始地址"=0, "读写标志"=0, "长度"=0}  # 信息帧
        w402 = T7 {"Current VI Reference"=refnum, "Close Panel on Exit?"=FALSE}  # Core
        n184 = property on="地检按钮" class="Bool (严格)"("Value"=w392) -> ()  [unwired: 2 in, 2 out]
        n185 = call <vilib>:"Write.vi"("Register name"="Beifen_on", "Register value"=w392) -> ()  [unwired: 11 in, 3 out]
        n186 = Bundle("Core"=w402, "传递队列输入"=w400, "信息帧"=w401, "主份控制指令"=w399, "备份控制指令"=w398, "notifier"=w396, "秒计数"=w395, "起始时间"=w394, "定时控制"=w393) -> (w404:T5)  [unwired: 1 in]
        n187 = call <vilib>:"Add State(s) to Queue__jki_lib_state_machine.vi"("State(s) in (\"\")"=w406) -> ("States Out"=w405:string)  [unwired: 14 in]
        n188 = property on="加计大小量程" class="RadioBtnsControl (严格)"("Value"=enum32{"小量程", "大量程"}."小量程" ("加计大小量程")) -> ()  [unwired: 2 in, 2 out]
      }
      frame "Data: Cleanup" {
        # "Cleanup any data and references, here.\n(this is called automatically, by the Macro: Exit)"
        n189 = Unbundle By Name(w407) -> ("Core.Current VI Reference"=w410:refnum<vi>)
        n190 = Close Reference(reference=w410, error in (no error)=w409) -> (error out=w408:errorcluster)
        n191 = call <vilib>:"Add State(s) to Queue__jki_lib_state_machine.vi"("State(s) in (\"\")"=w412) -> ("States Out"=w411:string)  [unwired: 14 in]
      }
      frame "---------- UI ----------" {
        # "Do not put any code in this frame.\n(It is a separator no-op. You can make a copy of this frame to create a new UI frame)"
        n192 = call <vilib>:"Add State(s) to Queue__jki_lib_state_machine.vi"("State(s) in (\"\")"=w416) -> ("States Out"=w415:string)  [unwired: 14 in]
      }
      frame "UI: Initialize" {
        w418 = u32 0
        # "Initialize the User Interface, here.\n(this is called automatically, by the Macro: Init)"
        n193 = property on="开始测量" class="Bool (严格)"("DisabledEnum"=T2."Enabled" ("禁用")) -> ()  [unwired: 2 in, 2 out]
        n194 = property on="停止测量" class="Bool (严格)"("DisabledEnum"=T2."Disabled and Grayed Out" ("禁用")) -> ()  [unwired: 2 in, 2 out]
        n195 = call <vilib>:"Write.vi"("Register name"="Packs_err_num_Beifen", "Register value"=w418) -> ()  [unwired: 11 in, 3 out]
        n196 = property on="正确帧计数" class="DigNum (严格)"("Value"=u16 0 ("脉冲  累计")) -> ()  [unwired: 2 in, 2 out]
        n197 = property on="错误帧计数" class="DigNum (严格)"("Value"=w418) -> ()  [unwired: 2 in, 2 out]
        n198 = call <vilib>:"Add State(s) to Queue__jki_lib_state_machine.vi"("State(s) in (\"\")"=w425) -> ("States Out"=w424:string)  [unwired: 14 in]
      }
      frame "UI: Cursor Set" {
        # "Argument"
        # "Set and Unset Cursor Busy.\n(Usage: \"UI: Cursor Set >> Busy|Idle\")"
        n199 = case shown="\"Idle\", 默认" w426 {
          tunnel: w428 -> [w433 w435]
          tunnel: [w432 w434] -> w427
          frame "Idle", Default {
            n200 = call <vilib>:"Unset Busy.vi"("error in (no error)"=w433) -> ("error out"=w432:errorcluster)  [unwired: 10 in]
          }
          frame "Busy" {
            n201 = call <vilib>:"Set Busy.vi"("error in (no error)"=w435) -> ("error out"=w434:errorcluster)  [unwired: 9 in, 1 out]
          }
        }
        n202 = call <vilib>:"Add State(s) to Queue__jki_lib_state_machine.vi"("State(s) in (\"\")"=w431) -> ("States Out"=w430:string)  [unwired: 14 in]
      }
      frame "UI: Front Panel State" {
        # "Set Front Panel Open or Closed\n(Usage: \"UI: Front Panel State >> Open|Close\")"
        n203 = disable-structure shown="启用" {
          disable-tunnel: w439 -> [w446 w469]
          disable-tunnel: [w445 w469] -> w438
          disable-tunnel: w437 -> [w444 _]
          disable-tunnel: w436 -> [w442 _]
          frame Disabled {
            # "Argument"
            n204 = Unbundle By Name(w444) -> ("Core.Current VI Reference"=w443:refnum<vi>)
            n205 = case shown="\"Open\", 默认" w442 {
              tunnel: w446 -> [w450 w463]
              tunnel: [w452 w464] -> w445
              tunnel: w443 -> [w451 w461]
              frame "Open", Default {
                n206 = property class="VI"(reference=w451, error in=w450) -> (reference out=w448:refnum<vi>, error out=w449:errorcluster, "Front Panel.Open"=w447:bool)
                n207 = case shown="假" w447 {
                  tunnel: [w455 w458] -> w452
                  tunnel: w449 -> [w454 w458]
                  tunnel: w448 -> [w453 _]
                  frame False {
                    n208 = invoke class="VI" method="FP.Open"(reference=w453, error in=w454, "Activate"=TRUE, "State"=T4."Standard") -> (error out=w455:errorcluster)  [unwired: 1 in, 4 out]
                  }
                  frame True {
                  }
                }
              }
              frame "Close" {
                n209 = property class="VI"(reference=w461, error in=w463) -> (reference out=w460:refnum<vi>, error out=w462:errorcluster, "Front Panel.Open"=w459:bool)
                n210 = case shown="真" w459 {
                  tunnel: [w465 w468] -> w464
                  tunnel: w462 -> [w465 w467]
                  tunnel: w460 -> [_ w466]
                  frame False {
                  }
                  frame True {
                    n211 = invoke class="VI" method="FP.Close"(reference=w466, error in=w467) -> (error out=w468:errorcluster)  [unwired: 1 in, 2 out]
                  }
                }
              }
            }
          }
          frame Enabled {
          }
        }
        n212 = call <vilib>:"Add State(s) to Queue__jki_lib_state_machine.vi"("State(s) in (\"\")"=w441) -> ("States Out"=w440:string)  [unwired: 14 in]
      }
      frame "---------- Macro ----------" {
        # "Do not put any code in this frame.\n(It is a separator no-op. You can make a copy of this frame to create a new Macro frame)"
        n213 = call <vilib>:"Add State(s) to Queue__jki_lib_state_machine.vi"("State(s) in (\"\")"=w473) -> ("States Out"=w472:string)  [unwired: 14 in]
      }
      frame "Macro: Initialize" {
        w474 = "Data: Initialize\nInitialize Core Data\nUI: Initialize\nUI: Front Panel State >> Open"  # Data: Initialize Initialize Core Data UI: Initialize UI: Front Panel State >> Open
        # "Initialization Macro\n(This is called once, when the VI starts)"
        n214 = call <vilib>:"Add State(s) to Queue__jki_lib_state_machine.vi"("State(s) in Front (\"\")"=w474, "State(s) in (\"\")"=w478) -> ("States Out"=w477:string)  [unwired: 13 in]
      }
      frame "Macro: Exit" {
        # "Exit Macro\n(This is called once, when the VI exits)"
        n215 = Unbundle By Name(w485) -> ("Core.Close Panel on Exit?"=w484:bool)
        n216 = Select(t="UI: Front Panel State >> Close", s=w484, f="") -> (s? t:f=w481:string)
        n217 = call <vilib>:"Add State(s) to Queue__jki_lib_state_machine.vi"("State(s) in (\"\")"=w481, "State(s) at Back (\"\")"="Data: Cleanup\nExit") -> ("States Out"=w479:string)  [unwired: 13 in]
        n218 = call <vilib>:"Add State(s) to Queue__jki_lib_state_machine.vi"("State(s) in Front (\"\")"=w479, "State(s) in (\"\")"=w488) -> ("States Out"=w487:string)  [unwired: 13 in]
      }
      frame "----------Request----------" {
        # "Template Separator\n(You can make a copy of, or modify, this frame)"
        n219 = call <vilib>:"Add State(s) to Queue__jki_lib_state_machine.vi"("State(s) in (\"\")"=w492) -> ("States Out"=w491:string)  [unwired: 14 in]
      }
      frame "Request:Write" {
        n220 = in-place {
          in-place-border: w496 -> [w502]
          in-place-border: [w501] -> w495
          in-place-border: w493 -> [w500]
          n221 = in-place-cluster #1(w497) -> ("传递队列输入"=w506:refnum<queue>, "信息帧"=w505:T6)
          n222 = in-place {
            in-place-border: w500 -> [w507]
            n223 = in-place-cluster #2(w505) -> ("数据"=w512:string)  [unwired: 5 out]
            n224 = in-place-cluster #2("数据帧名称"=w507, "数据"=w512, "备用操作符"=TRUE, "起始地址"=0, "读写标志"=1, "长度"=0) -> (w504:T6)
          }
          n225 = Enqueue Element(queue=w506, element=w504, error in (no error)=w502) -> (queue out=w503:refnum<queue>, error out=w501:errorcluster)  [unwired: 1 in, 1 out]
          n226 = in-place-cluster #1("传递队列输入"=w503, "信息帧"=w504) -> (w494:T5)
        }
        n227 = call <vilib>:"Add State(s) to Queue__jki_lib_state_machine.vi"("State(s) in (\"\")"=w499) -> ("States Out"=w498:string)  [unwired: 14 in]
      }
      frame "Config:Write" {
        n228 = in-place {
          in-place-border: w516 -> [w522]
          in-place-border: [w521] -> w515
          in-place-border: w513 -> [w520]
          n229 = in-place-cluster #3(w517) -> ("传递队列输入"=w526:refnum<queue>, "信息帧"=w525:T6)
          n230 = in-place {
            in-place-border: w520 -> [w527]
            n231 = in-place-cluster #4(w525) -> ("数据"=w532:string)  [unwired: 5 out]
            n232 = in-place-cluster #4("数据帧名称"=w527, "数据"=w532, "备用操作符"=TRUE, "起始地址"=0, "读写标志"=2, "长度"=0) -> (w524:T6)
          }
          n233 = Enqueue Element(queue=w526, element=w524, error in (no error)=w522) -> (queue out=w523:refnum<queue>, error out=w521:errorcluster)  [unwired: 1 in, 1 out]
          n234 = in-place-cluster #3("传递队列输入"=w523, "信息帧"=w524) -> (w514:T5)
        }
        n235 = call <vilib>:"Add State(s) to Queue__jki_lib_state_machine.vi"("State(s) in (\"\")"=w519) -> ("States Out"=w518:string)  [unwired: 14 in]
      }
      frame "Request:OPEN1553B" {
        n236 = in-place {
          in-place-border: w536 -> [w543]
          in-place-border: [w542] -> w535
          in-place-border: w533 -> [w540]
          n237 = in-place-cluster #5(w537) -> ("传递队列输入"=w546:refnum<queue>, "信息帧"=w541:T6)
          n238 = in-place {
            in-place-border: w540 -> [w547]
            n239 = in-place-cluster #6(w541) -> ()  [unwired: 6 out]
            n240 = in-place-cluster #6("数据帧名称"=w547, "数据"="$B\n", "备用操作符"=TRUE, "起始地址"=0, "读写标志"=1, "长度"=0) -> (w545:T6)
          }
          n241 = Enqueue Element(queue=w546, element=w545, error in (no error)=w543) -> (queue out=w544:refnum<queue>, error out=w542:errorcluster)  [unwired: 1 in, 1 out]
          n242 = in-place-cluster #5("传递队列输入"=w544, "信息帧"=w541) -> (w534:T5)
        }
        n243 = call <vilib>:"Add State(s) to Queue__jki_lib_state_machine.vi"("State(s) in (\"\")"=w539) -> ("States Out"=w538:string)  [unwired: 14 in]
      }
      frame "Request:Close1553B" {
        n244 = in-place {
          in-place-border: w555 -> [w564]
          in-place-border: [w563] -> w554
          n245 = in-place-cluster #7(w556) -> ("传递队列输入"=w566:refnum<queue>, "信息帧"=w560:T6)
          n246 = in-place {
            n247 = in-place-cluster #8(w560) -> ()  [unwired: 6 out]
            n248 = in-place-cluster #8("数据帧名称"="1553B_CMD", "数据"="$", "备用操作符"=TRUE, "起始地址"=0, "读写标志"=1, "长度"=0) -> (w565:T6)
          }
          n249 = in-place {
            n250 = in-place-cluster #9(w560) -> ()  [unwired: 6 out]
            n251 = in-place-cluster #9("数据帧名称"="1553B_CMD", "数据"="$Z\n", "备用操作符"=TRUE, "起始地址"=0, "读写标志"=1, "长度"=0) -> (w561:T6)
          }
          n252 = Enqueue Element(queue=w566, element=w565, error in (no error)=w564) -> (queue out=w562:refnum<queue>, error out=w563:errorcluster)  [unwired: 1 in, 1 out]
          n253 = Enqueue Element(queue=w562, element=w561) -> (queue out=w559:refnum<queue>)  [unwired: 2 in, 2 out]
          n254 = in-place-cluster #7("传递队列输入"=w559, "信息帧"=w560) -> (w553:T5)
        }
        n255 = call <vilib>:"Add State(s) to Queue__jki_lib_state_machine.vi"("State(s) in (\"\")"=w558) -> ("States Out"=w557:string)  [unwired: 14 in]
      }
      frame "Request:Read" {
        n256 = in-place {
          in-place-border: w581 -> [w586]
          in-place-border: [w585] -> w580
          n257 = in-place-cluster #10(w582) -> ("传递队列输入"=w590:refnum<queue>, "信息帧"=w589:T6)
          n258 = in-place {
            n259 = in-place-cluster #11(w589) -> ("数据"=w595:string)  [unwired: 5 out]
            n260 = in-place-cluster #11("数据帧名称"="GNSS1", "数据"=w595, "备用操作符"=TRUE, "起始地址"=0, "读写标志"=0, "长度"=0) -> (w588:T6)
          }
          n261 = Enqueue Element(queue=w590, element=w588, error in (no error)=w586) -> (queue out=w587:refnum<queue>, error out=w585:errorcluster)  [unwired: 1 in, 1 out]
          n262 = in-place-cluster #10("传递队列输入"=w587, "信息帧"=w588) -> (w579:T5)
        }
        n263 = call <vilib>:"Add State(s) to Queue__jki_lib_state_machine.vi"("State(s) in (\"\")"=w584) -> ("States Out"=w583:string)  [unwired: 14 in]
      }
      frame "----------Usr----------" {
        # "Template Separator\n(You can make a copy of, or modify, this frame)"
        n264 = call <vilib>:"Add State(s) to Queue__jki_lib_state_machine.vi"("State(s) in (\"\")"=w600) -> ("States Out"=w599:string)  [unwired: 14 in]
      }
      frame "Exit:all" {
        n265 = call <vilib>:"Add State(s) to Queue__jki_lib_state_machine.vi"("State(s) in Front (\"\")"="Macro: Exit", "State(s) in (\"\")"=w605) -> ("States Out"=w604:string)  [unwired: 13 in]
      }
      frame "Usr:Frame-init" {
        n266 = in-place {
          n267 = in-place-cluster #12(w607) -> ()  [unwired: 1 out]
          n268 = Initialize Array(u8 0 ("元素"), 218 ("维数大小")) -> (w614:u8[])
          n269 = Replace Array Subset(array=w614, new element=u8[] [170, 85, 218, 0], index=0 ("索引")) -> (w611:u8[])
          n270 = Byte Array To String(unsigned byte array=w611) -> (string=w617:string)
          n271 = in-place-cluster #12("信息帧.数据"=w617) -> (w606:T5)
        }
        n272 = call <vilib>:"Add State(s) to Queue__jki_lib_state_machine.vi"("State(s) in (\"\")"=w610) -> ("States Out"=w609:string)  [unwired: 14 in]
      }
      frame "Usr:Frame-set" {
        n273 = disable-structure shown="禁用" {
          disable-tunnel: ["Request:Write" ("State(s) in Front (\"\")") _] -> w619
          frame Disabled {
          }
          frame Enabled {
          }
        }
        n274 = call <vilib>:"Add State(s) to Queue__jki_lib_state_machine.vi"("State(s) in (\"\")"=w622, "State(s) at Back (\"\")"=w619) -> ("States Out"=w621:string)  [unwired: 13 in]
      }
      frame "Usr:Update_timestap" {
        n275 = Get Date/Time In Seconds() -> (seconds since 1Jan1904=w638:timestamp)
        n276 = Seconds To Date/Time(time stamp (now)=w638) -> (date time rec=w630:T1)  [unwired: 1 in]
        n277 = Unbundle By Name(w630) -> ("时"=w631:i32, "分"=w634:i32, "秒"=w624:i32)
        n278 = Multiply(x=w631, y=60) -> (x*y=w633:i32)
        n279 = Add(x=w633, y=w634) -> (x+y=w635:i32)
        n280 = Multiply(x=w635, y=60) -> (x*y=w637:i32)
        n281 = Add(x=w637, y=w624) -> (x+y=w629:i32)
        n282 = To Quad Integer(1:w629) -> (0:w628:i64)
        n283 = call <vilib>:"Add State(s) to Queue__jki_lib_state_machine.vi"("State(s) in (\"\")"=w640) -> ("States Out"=w639:string)  [unwired: 14 in]
        n284 = Bundle By Name(cluster=w627, "起始时间"=w628) -> (w626:T5)
      }
    }
  }
  n285 = while {
    tunnel: "notifier" -> [w646]
    stop <- w645 stop-if-true
    n286 = call "stop_message.vi"("notifier"=w646) -> ("Exit？"=w645:bool)  [unwired: 9 in, 1 out]
    n287 = call <vilib>:"Read.vi"("Register name"="Beifen_on") -> ("Register value"=w643:variant)  [unwired: 11 in, 3 out]
    n288 = call-poly <vilib>:"Convert.vi"("Register value in"=w643) -> ("Register value out"=w642:bool)  [unwired: 13 in, 1 out]
    n289 = Wait (ms)(milliseconds to wait=u32 100 ("等待时间（毫秒）")) -> ()  [unwired: 1 out]
    n290 = case shown="真" w642 {
      frame False {
      }
      frame True {
        n291 = call <vilib>:"Read.vi"("Register name"="Run_mode") -> ("Register value"=w656:variant)  [unwired: 11 in, 3 out]
        n292 = call <vilib>:"Read.vi"("Register name"="Packs_err_num_Beifen") -> ("Register value"=w650:variant)  [unwired: 11 in, 3 out]
        n293 = call-poly <vilib>:"Convert.vi"("Register value in"=w656) -> ("Register value out"=w654:u8)  [unwired: 13 in, 1 out]
        n294 = call <vilib>:"Read.vi"("Register name"="Packs_ok_num_Beifen") -> ("Register value"=w649:variant)  [unwired: 11 in, 3 out]
        n295 = call-poly <vilib>:"Convert.vi"("Register value in"=w650) -> ("Register value out"=→"错误帧计数":u32)  [unwired: 13 in, 1 out]
        n296 = call-poly <vilib>:"Convert.vi"("Register value in"=w649) -> ("Register value out"=→"正确帧计数":u32)  [unwired: 13 in, 1 out]
        n297 = call <vilib>:"Read.vi"("Timeout"=1, "Register name"="1553BBeiFenRecv_stat") -> ("Register value"=w657:variant, "Register value read?"=w653:bool)  [unwired: 10 in, 2 out]
        n298 = case shown="真" w653 {
          tunnel: w657 -> [_ w669]
          tunnel: w654 -> [_ w668]
          frame False {
          }
          frame True {
            n299 = call "state_sep.vi"("Register value"=w669, "MODE"=w668) -> ("G1陀螺脉冲数"=→"主份G1陀螺脉冲数":dbl, "G2陀螺脉冲数"=→"主份G2陀螺脉冲数":dbl, "G3陀螺脉冲数"=→"主份G3陀螺脉冲计数":dbl, "A1加速度计脉冲数"=→"主份A1加速度计脉冲计数":dbl, "A2加速度计脉冲数"=→"主份A2加速度计脉冲计数":dbl, "温度"=→"温度":string, "脉冲计数"=→"脉冲计数":string, "A3加速度计脉冲数"=→"主份A3加速度计脉冲计数":dbl)  [unwired: 17 in, 1 out]
          }
        }
      }
    }
  }
